vi "Servo MSMT GSM Set RF WFM Parameters.vi"(8 "error in (no error)":errorcluster, 10 "Step In":refnum<k7>, 11 "Servo MSMT in":refnum<class "Servo MSMT.lvclass">) -> (0 "error out":errorcluster, 2 "Step Out":refnum<k7>, 3 "Servo MSMT out":refnum<class "Servo MSMT.lvclass">)   [LabVIEW 2018, in "Servo MSMT.lvlib" / "Servo MSMT.lvclass"]
uses:
  Servo MSMT.lvclass
  C:/Sequence Automation/Plugins/Measurement Interface.lvlibp/Measurement Interface.lvclass
  Plugins/Measurement Interface.lvlibp/Private Methods/Measurement Parameters/Read Measurement Parameters.vi
  Plugins/String Database.lvlibp/String Database.lvclass
  Plugins/TestStand API Tools (TSAT).lvlibp/Step Actions/TSAT Step Actions.lvlib
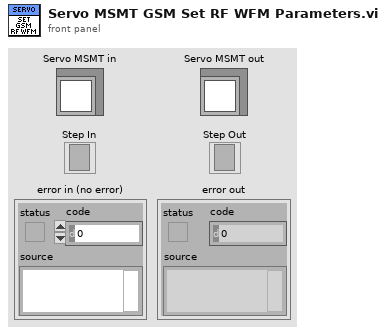
[diagram p1: front panel]
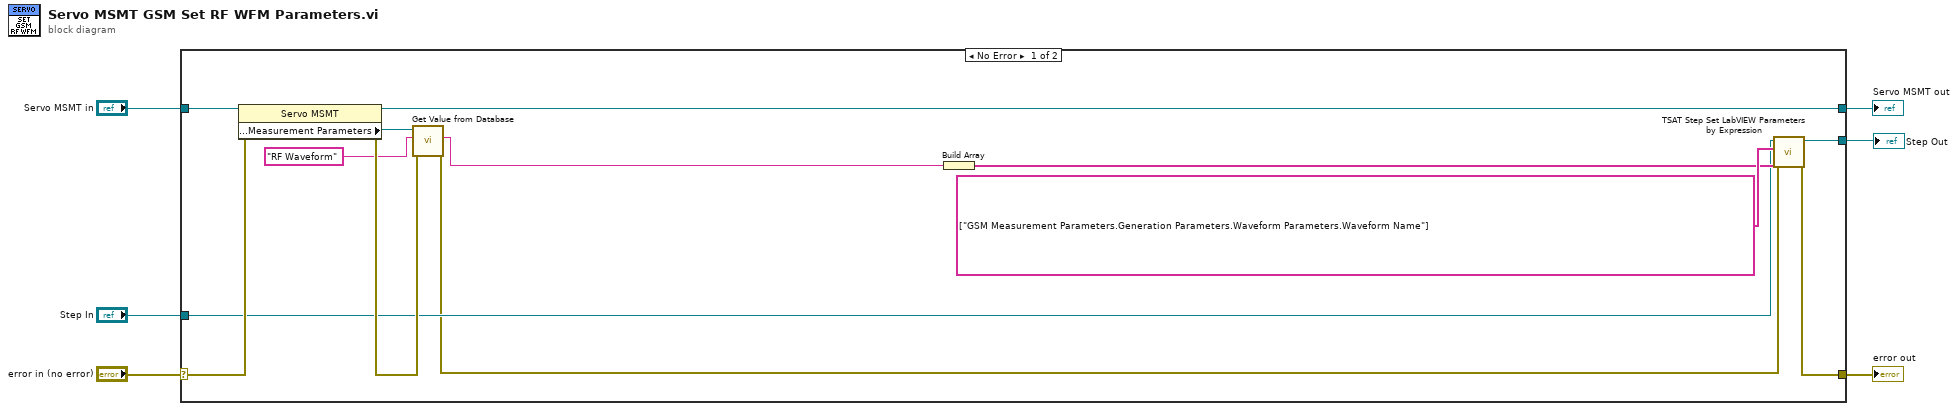
[diagram p0: block diagram]
diagram:
  n1 = case shown="No Error" "error in (no error)" {
    selector: "error in (no error)" -> [w19 w22]
    tunnel: [w18 w22] -> w5
    tunnel: [w9 w21] -> w3
    tunnel: "Servo MSMT in" -> [w17 w21]
    tunnel: [w11 w20] -> w2
    tunnel: "Step In" -> [w10 w20]
    frame No Error {
      n2 = property class="Servo MSMT"(reference=w17, error in=w19) -> (reference out=w9:refnum<class "Servo MSMT.lvclass">, error out=w15:errorcluster, "Protected Methods:Measurement Parameters"=w16:refnum<class "String Database.lvclass">)
      n3 = call "Get Value from Database.vi"("error in (no error)"=w15, "Entry Name"="RF Waveform", "Message in"=w16) -> ("error out"=w7:errorcluster, "Entry Value"=w8:string)  [unwired: 5 in, 2 out]
      n4 = Build Array(w8) -> (w12:string[])
      n5 = call "TSAT Step Set LabVIEW Parameters by Expression.vi"("Error In"=w7, "Value Expressions"=w12, "Parameters to Set"=string[] ["GSM Measurement Parameters.Generation Parameters.Waveform Parameters.Waveform Name"], "Step In"=w10) -> ("Error Out"=w18:errorcluster, "Step Out"=w11:refnum<k7>)  [unwired: 6 in]
    }
    frame Error {
    }
  }
  "error out" <- w5
  "Servo MSMT out" <- w3
  "Step Out" <- w2
